vi "Scheduler (SubVI).vi"(2 "error in (no error)":errorcluster, 3 "queue in":refnum<queue>, 4 "is_running":refnum<vi>, 5 "stop":refnum<vi>) -> (0 "error out":errorcluster)   [LabVIEW 2016]
uses:
  global/Config_Infos.vi
panel:
  in  "start added to queue?":bool
  out "current time":timestamp
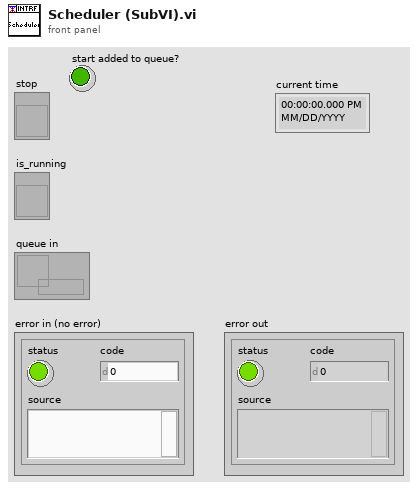
[diagram p1: front panel]
types:
  T1 = typedef "LVDateTimeRec.ctl" = cluster{"fractional second":dbl, "second":i32, "minute":i32, "hour":i32, "day of month":i32, "month":i32, "year":i32, "day of week":i32, "day of year":i32, "DST":i32}
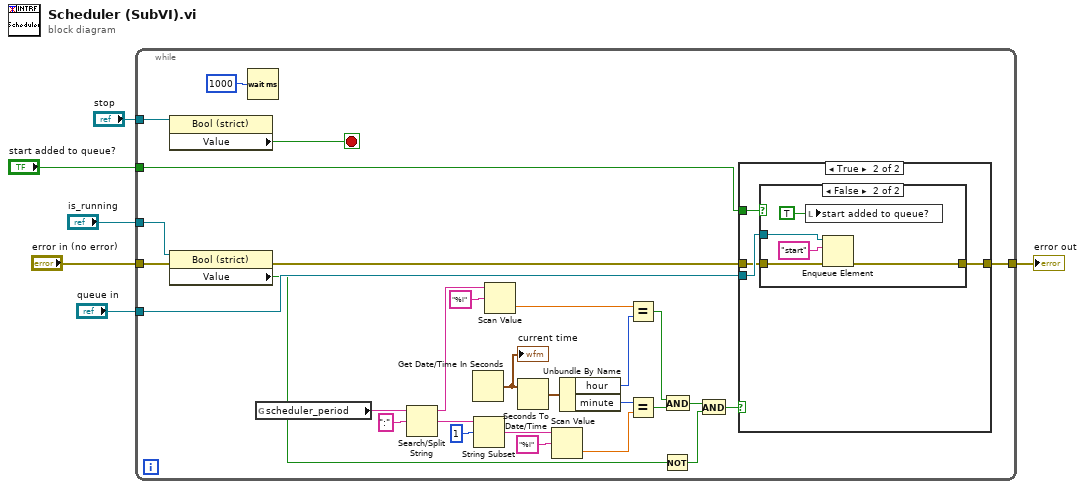
[diagram p0: block diagram]
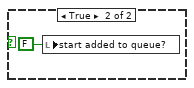
[diagram p3: hidden frame]
diagram:
  n1 = while {
    tunnel: "queue in" -> [w35]
    tunnel: "error in (no error)" -> [w22]
    tunnel: [w33] -> w6
    tunnel: "stop" -> [w29]
    tunnel: "is_running" -> [w28]
    tunnel: "start added to queue?" -> [w7]
    stop <- w32 stop-if-true
    n2 = property class="Bool (strict)"(reference=w29) -> ("Value"=w32:bool)  [unwired: 1 in, 2 out]
    n3 = property class="Bool (strict)"(reference=w28, error in=w22) -> (error out=w23:errorcluster, "Value"=w31:bool)  [unwired: 1 out]
    n4 = Wait (ms)(milliseconds to wait=u32 1000) -> ()  [unwired: 1 out]
    n5 = global read "Config_Infos.vi" "scheduler_period"() -> (w25:string)
    n6 = Search/Split String(string=w25, search string/char (-)=":") -> (substring before match=w21:string, match + rest of string=w19:string)  [unwired: 1 in, 1 out]
    n7 = Get Date/Time In Seconds() -> (seconds since 1Jan1904=w27:timestamp)
    "current time" <- w27
    n8 = String Subset(string=w19, offset (0)=1) -> (substring=w16:string)  [unwired: 1 in]
    n9 = Scan Value(string=w21, format string="%i") -> (value=w9:dbl)  [unwired: 1 in, 1 out]
    n10 = Seconds To Date/Time(time stamp (now)=w27) -> (date time rec=w26:T1)  [unwired: 1 in]
    n11 = Scan Value(string=w16, format string="%i") -> (value=w14:dbl)  [unwired: 1 in, 1 out]
    n12 = Unbundle By Name(w26) -> ("hour"=w10:i32, "minute"=w15:i32)
    n13 = Equal?(x=w9, y=w10) -> (x = y?=w13:bool)
    n14 = Equal?(x=w15, y=w14) -> (x = y?=w12:bool)
    n15 = Not(x=w31) -> (.not. x?=w34:bool)
    n16 = And(x=w13, y=w12) -> (x .and. y?=w11:bool)
    n17 = And(x=w11, y=w34) -> (x .and. y?=w8:bool)
    n18 = case shown="True" w8 {
      tunnel: w35 -> [_ w42]
      tunnel: [w37 w41] -> w33
      tunnel: w23 -> [w37 w40]
      tunnel: w7 -> [w36 w39]
      frame False {
        n19 = case shown="False" w36 {
          frame False {
          }
          frame True {
            n20 = local write "start added to queue?"(FALSE ("start added to queue?")) -> ()
          }
        }
      }
      frame True {
        n21 = case shown="False" w39 {
          tunnel: w42 -> [_ w48]
          tunnel: [w43 w47] -> w41
          tunnel: w40 -> [w43 w45]
          frame True {
          }
          frame False {
            n22 = local write "start added to queue?"(TRUE ("start added to queue?")) -> ()
            n23 = Enqueue Element(queue=w48, element="start", error in (no error)=w45) -> (error out=w47:errorcluster)  [unwired: 1 in, 2 out]
          }
        }
      }
    }
  }
  "error out" <- w6
